vi "getPoints.vi"(0 "reference":refnum<class "StateTransitionEdge.lvclass">, 5 "error in (no error)":errorcluster) -> (14 "reference out":refnum<class "StateTransitionEdge.lvclass">, 15 "points":T1[](array[typedef]) {"y" format="%.2f"; "x" format="%.2f"}, 19 "error out":errorcluster)   [LabVIEW 2016, in "StateTransitionEdge.lvclass"]
doc: "Abstract getPoints"
uses:
  <resource>/Framework/Providers/Open_GDS/UML/StateTransitionEdge_class/StateTransitionEdge.lvclass
  C:/Program Files (x86)/National Instruments/LabVIEW 2016/resource/Framework/Providers/Open_GDS/UML/ClassRelationshipEdge_class/ClassRelationshipEdge.lvclass
  C:/Program Files (x86)/National Instruments/LabVIEW 2016/resource/Framework/Providers/Open_GDS/UML/AbstractEdge_class/AbstractEdge.lvclass
  <resource>/Framework/Providers/Open_GDS/UML/General/Point/Point Point2D.ctl
  <resource>/Framework/Providers/Open_GDS/UML/BentStyle_class/BentStyle.lvclass
  <resource>/Framework/Providers/Open_GDS/UML/ClassRelationshipEdge_class/ClassRelationshipEdge.lvclass
  <resource>/Framework/Providers/Open_GDS/UML/AbstractNode_class/AbstractNode.lvclass
  <resource>/Framework/Providers/Open_GDS/UML/AbstractEdge_class/AbstractEdge.lvclass
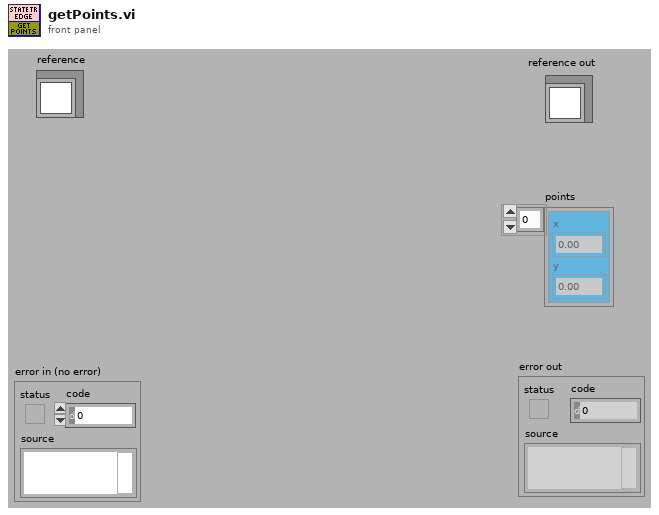
[diagram p1: front panel]
types:
  T1 = typedef "Point Point2D.ctl" = cluster{"x":dbl, "y":dbl}
  T2 = typedef "ClassRelationshipEdge.lvclass/ObjectAttributes.ctl" = cluster{"bentStyleRef":refnum<class "BentStyle.lvclass">, "startConnectionOffset":cluster{"x":i32, "y":i32}, "endConnectionOffset":cluster{"x":i32, "y":i32}, "MidLineOffset":cluster{"x":i32, "y":i32}, "DepClass":T3}
  T3 = typedef "ReversedEngineering_ViDependencyDetailsType.ctl" = cluster{"ThisVIs/Ctls":path[], "Dependent_VIs/Ctls":path[]}
  T4 = typedef "AbstractEdge.lvclass/ObjectAttributes.ctl" = cluster{"start":refnum<class "AbstractNode.lvclass">, "end":refnum<class "AbstractNode.lvclass">}
  T5 = typedef "BentStyle.lvclass/BentStyleType.ctl" = enum16{"STRAIGHT", "HV", "VH", "HVH", "VHV", "ARC"}
  T6 = typedef "Rectangle Rectangle2D.ctl" = cluster{"x":dbl, "y":dbl, "width":dbl, "height":dbl}
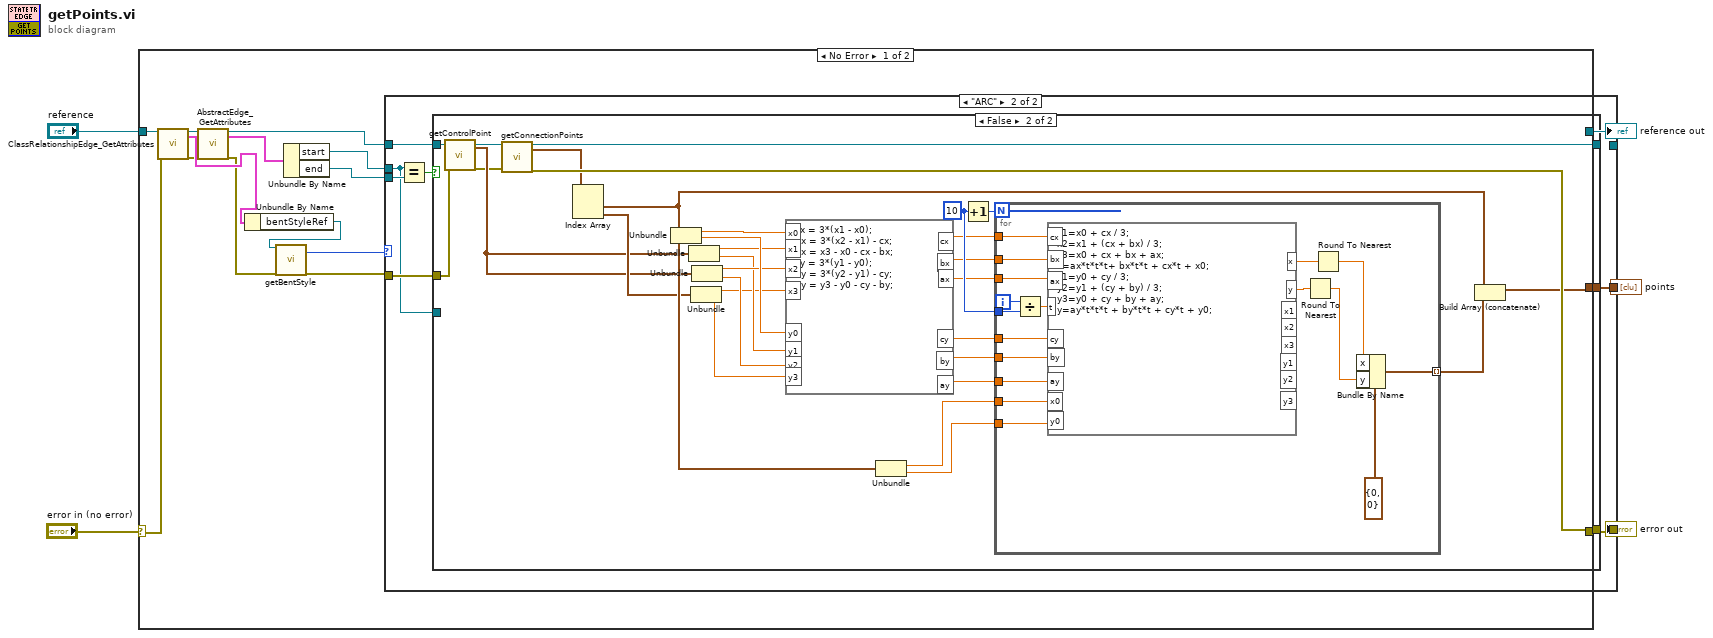
[diagram p0: block diagram]
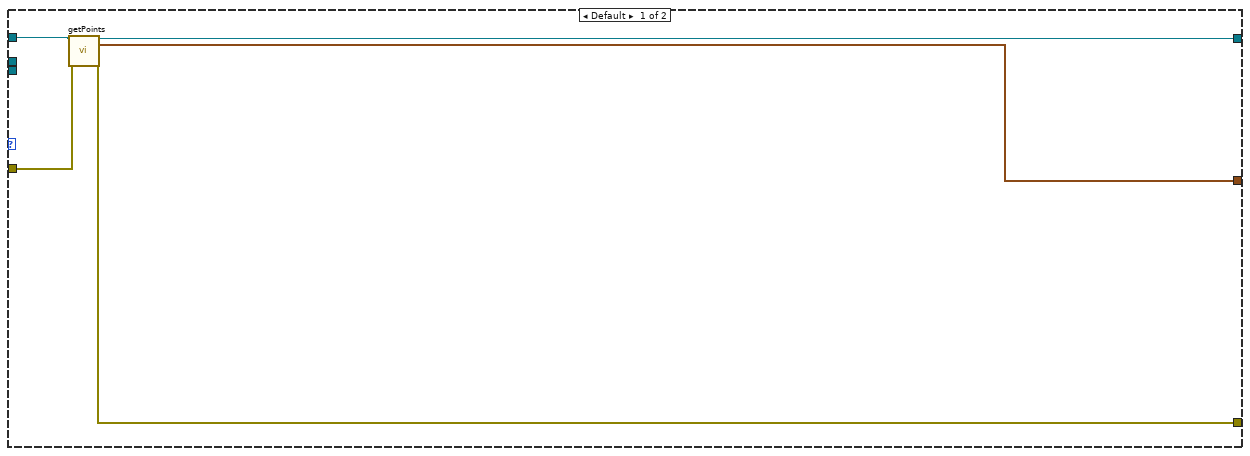
[diagram p2: hidden frame]
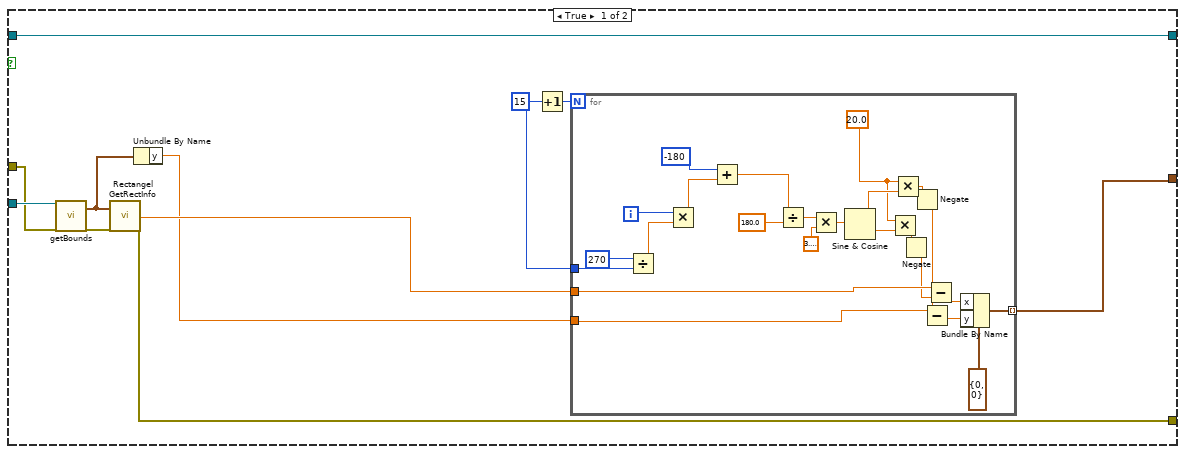
[diagram p3: hidden frame]
diagram:
  n1 = case shown="No Error" "error in (no error)" {
    selector: "error in (no error)" -> [w14 w116]
    tunnel: "reference" -> [w18 w117]
    tunnel: [w21 w116] -> w4
    tunnel: [w20 w117] -> w3
    tunnel: [w19 _] -> w1
    frame No Error {
      n2 = call <resource>:"ClassRelationshipEdge_GetAttributes.vi"("reference in"=w18, "error in (no error)"=w14) -> ("reference out"=w10:refnum<class "StateTransitionEdge.lvclass">, "Data"=w11:T2, "error out"=w9:errorcluster)  [unwired: 14 in, 1 out]
      n3 = call <resource>:"AbstractEdge_GetAttributes.vi"("reference in"=w10, "error in (no error)"=w9) -> ("reference out"=w7:refnum<class "StateTransitionEdge.lvclass">, "Data"=w6:T4, "error out"=w8:errorcluster)  [unwired: 14 in, 1 out]
      n4 = Unbundle By Name(w11) -> ("bentStyleRef"=w17:refnum<class "BentStyle.lvclass">)
      n5 = call-dynamic "getBentStyle.vi"("reference"=w17, "error in (no error)"=w8) -> ("bentStyle"=w16:T5, "error out"=w15:errorcluster)  [unwired: 15 in, 1 out]
      n6 = Unbundle By Name(w6) -> ("start"=w13:refnum<class "AbstractNode.lvclass">, "end"=w12:refnum<class "AbstractNode.lvclass">)
      n7 = case shown="\"ARC\"" w16 {
        tunnel: [w23 w34] -> w21
        tunnel: [w25 w33] -> w20
        tunnel: [w24 w32] -> w19
        tunnel: w7 -> [w26 w31]
        tunnel: w15 -> [w22 w30]
        tunnel: w13 -> [_ w27]
        tunnel: w12 -> [_ w29]
        frame Default {
          n8 = call-parent "getPoints.vi"("reference"=w26, "error in (no error)"=w22) -> ("reference out"=w25:refnum<class "StateTransitionEdge.lvclass">, "points"=w24:T1[], "error out"=w23:errorcluster)  [unwired: 15 in]
        }
        frame "ARC" {
          n9 = Equal?(x=w27, y=w29) -> (x = y?=w28:bool)
          n10 = case shown="False" w28 {
            tunnel: [w37 w98] -> w34
            tunnel: [w45 w97] -> w33
            tunnel: [w43 w96] -> w32
            tunnel: w31 -> [w45 w71]
            tunnel: w30 -> [w41 w70]
            tunnel: w27 -> [w42 _]
            frame True {
              w40 = 15
              n11 = call-dynamic "getBounds.vi"("reference"=w42, "error in (no error)"=w41) -> ("bounds"=w36:T6, "error out"=w44:errorcluster)  [unwired: 15 in, 1 out]
              n12 = call <resource>:"Rectangel GetRectInfo.vi"("bounds"=w36, "error in (no error)"=w44) -> ("maxX"=w38:dbl, "error out"=w37:errorcluster)  [unwired: 16 out]
              n13 = Unbundle By Name(w36) -> ("y"=w35:dbl)
              n14 = Increment(x=w40) -> (x+1=w39:i32)
              n15 = for {
                N: w39 -> [_]
                tunnel: [w68] -> w43 mode=indexing
                tunnel: w40 -> [w64]
                tunnel: w35 -> [w50]
                tunnel: w38 -> [w51]
                i -> [w66]
                w52 = 20.0 ("y")
                n16 = Divide(x=270, y=w64) -> (x/y=w63:dbl)
                n17 = Multiply(x=w66, y=w63) -> (x*y=w62:dbl)
                n18 = Add(x=-180, y=w62) -> (x+y=w57:dbl)
                n19 = Divide(x=w57, y=180.0) -> (x/y=w58:dbl)
                n20 = Multiply(x=w58, y=3.141592653589793) -> (x*y=w60:dbl)
                n21 = Sine & Cosine(0:w60) -> (1:w56:dbl, 2:w53:dbl)
                n22 = Multiply(x=w52, y=w53) -> (x*y=w48:dbl)
                n23 = Multiply(x=w52, y=w56) -> (x*y=w49:dbl)
                n24 = Negate(x=w48) -> (-x=w46:dbl)
                n25 = Negate(x=w49) -> (-x=w47:dbl)
                n26 = Subtract(x=w50, y=w47) -> (x-y=w55:dbl)
                n27 = Subtract(x=w51, y=w46) -> (x-y=w54:dbl)
                n28 = Bundle By Name(cluster=cluster{"x":i16, "y":i16} {"x"=0, "y"=0} ("end point"), "x"=w54, "y"=w55) -> (w68:cluster{"x":i16, "y":i16})
              }
            }
            frame False {
              w92 = 10
              n29 = call <resource>:"getControlPoint.vi"("reference"=w71, "error in (no error)"=w70) -> ("reference out"=w97:refnum<class "StateTransitionEdge.lvclass">, "point"=w73:T1, "error out"=w72:errorcluster)  [unwired: 15 out]
              n30 = call-dynamic "getConnectionPoints.vi"("reference"=w97, "error in (no error)"=w72) -> ("line"=w76:T1[], "error out"=w98:errorcluster)  [unwired: 15 in, 1 out]
              n31 = Index Array(array=w76) -> (element #1=w75:T1, element #2=w74:T1)  [unwired: 2 in]
              n32 = Unbundle(w75) -> ("x"=w87:dbl, "y"=w86:dbl)
              n33 = Unbundle(w73) -> ("x"=w85:dbl, "y"=w82:dbl)
              n34 = Unbundle(w74) -> ("x"=w78:dbl, "y"=w83:dbl)
              n35 = Unbundle(w73) -> ("x"=w84:dbl, "y"=w81:dbl)
              n36 = formula code="cx = 3*(x1 - x0);\nbx = 3*(x2 - x1) - cx;\nax = x3 - x0 - cx - bx;\ncy = 3*(y1 - y0);\nby = 3*(y2 - y1) - cy;\nay = y3 - y0 - cy - by;"("x0"=w87, "x1"=w85, "x2"=w84, "x3"=w78, "y0"=w86, "y1"=w82, "y2"=w81, "y3"=w83) -> ("cx"=w88:dbl, "bx"=w89:dbl, "ax"=w90:dbl, "cy"=w93:dbl, "by"=w94:dbl, "ay"=w95:dbl)
              n37 = Unbundle(w75) -> ("x"=w80:dbl, "y"=w79:dbl)
              n38 = Increment(x=w92) -> (x+1=w91:i32)
              n39 = for {
                N: w91 -> [_]
                tunnel: w88 -> [w115]
                tunnel: w89 -> [w114]
                tunnel: w90 -> [w113]
                tunnel: w92 -> [w111]
                tunnel: w93 -> [w104]
                tunnel: w94 -> [w103]
                tunnel: w95 -> [w102]
                tunnel: w80 -> [w101]
                tunnel: w79 -> [w100]
                tunnel: [w99] -> w77 mode=indexing
                i -> [w112]
                n40 = Divide(x=w112, y=w111) -> (x/y=w110:dbl)
                n41 = formula code="x1=x0 + cx / 3;\nx2=x1 + (cx + bx) / 3;\nx3=x0 + cx + bx + ax;\nx=ax*t*t*t+ bx*t*t + cx*t + x0;\ny1=y0 + cy / 3;\ny2=y1 + (cy + by) / 3;\ny3=y0 + cy + by + ay;\ny=ay*t*t*t + by*t*t + cy*t + y0;"("cx"=w115, "bx"=w114, "ax"=w113, "t"=w110, "cy"=w104, "by"=w103, "ay"=w102, "x0"=w101, "y0"=w100) -> ("x"=w108:dbl, "y"=w107:dbl)  [unwired: 6 out]
                n42 = Round To Nearest(number=w107) -> (nearest integer value=w105:dbl)
                n43 = Round To Nearest(number=w108) -> (nearest integer value=w106:dbl)
                n44 = Bundle By Name(cluster=cluster{"x":i16, "y":i16} {"x"=0, "y"=0} ("end point"), "x"=w106, "y"=w105) -> (w99:cluster{"x":i16, "y":i16})
              }
              n45 = Build Array (concatenate)(w75, w77) -> (w96:T1[])
            }
          }
        }
      }
    }
    frame Error {
    }
  }
  "reference out" <- w3
  "error out" <- w4
  "points" <- w1
